vi "Read Frame.vi"(8 "error in (no error)":errorcluster caption="entrée d'erreur (pas d'erreur)", 11 "Class Camera IV3-500CA (Default) en Entrée":refnum<class "Class Pattern Matching (Default).lvclass">) -> (0 "error out":errorcluster caption="sortie d'erreur", 3 "Class Camera IV3-500CA (Default) en Sortie":refnum<class "Class Pattern Matching (Default).lvclass">)   [LabVIEW 2020, in "Library Instrument & Equipement.lvlib" / "Library Camera.lvlib" / "Class Pattern Matching (Default).lvclass"]
uses:
  Class Pattern Matching (Default).lvclass
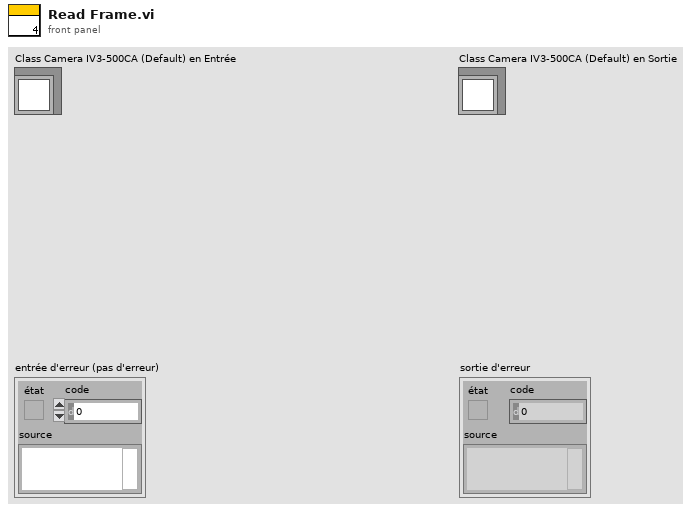
[diagram p1: front panel]
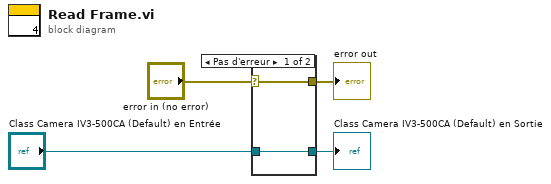
[diagram p0: block diagram]
diagram:
  n1 = case shown="Pas d'erreur" "error in (no error)" {
    selector: "error in (no error)" -> [w5 w8]
    tunnel: [w5 w8] -> w3
    tunnel: [w6 w7] -> w1
    tunnel: "Class Camera IV3-500CA (Default) en Entrée" -> [w6 w7]
    frame No Error {
    }
    frame Error {
    }
  }
  "error out" <- w3
  "Class Camera IV3-500CA (Default) en Sortie" <- w1
